vi "atpVI.vi"() -> ()   [LabVIEW 2013]
panel:
  in  "elbow":dbl(slide) scale=0.0..130.0
  in  "slew":dbl(slide) scale=0.0..120.0
  in  "shoulder":dbl(slide) scale=0.0..90.0
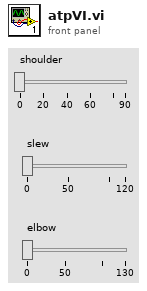
[diagram p1: front panel]
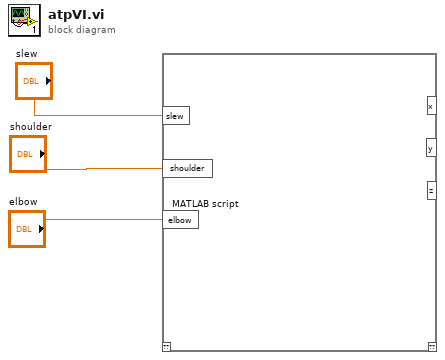
[diagram p0: block diagram]
diagram:
  n1 = script code="MATLAB script" ("Script Node")("slew"="slew", "shoulder"="shoulder", "elbow"="elbow") -> ()  [unwired: 1 in, 4 out]
